vi "route.vi"() -> ()   [LabVIEW 2014]
uses:
  <vilib>/Utility/sysdir.llb/System Directory Type.ctl
  <vilib>/httpClient/LabVIEWHTTPClient.lvlib
panel:
  out "full/연료":i32
  out "time/시간":dbl
  in  "도움말":bool
  in  "피드백":bool
  in  "저장 경로":path
  out "Distance":string="0"
  in  "?":bool
  in  "?":bool
  in  "?":bool
  out "x fmc 플랜":string
  out "FMS 플랜":string
  in  "Destination":string
  in  "departure":string
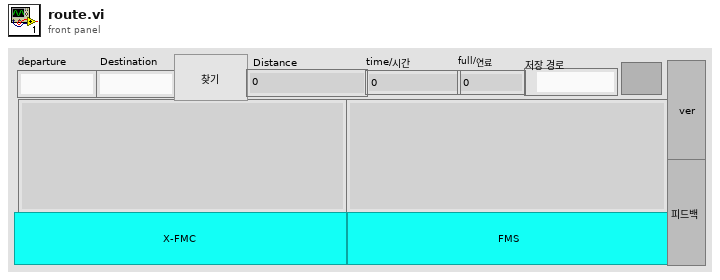
[diagram p1: front panel]
types:
  T1 = enum16{"open", "replace", "create", "open or create", "replace or create", "replace or create with confirmation"}
  T2 = typedef "System Directory Type.ctl" = i32
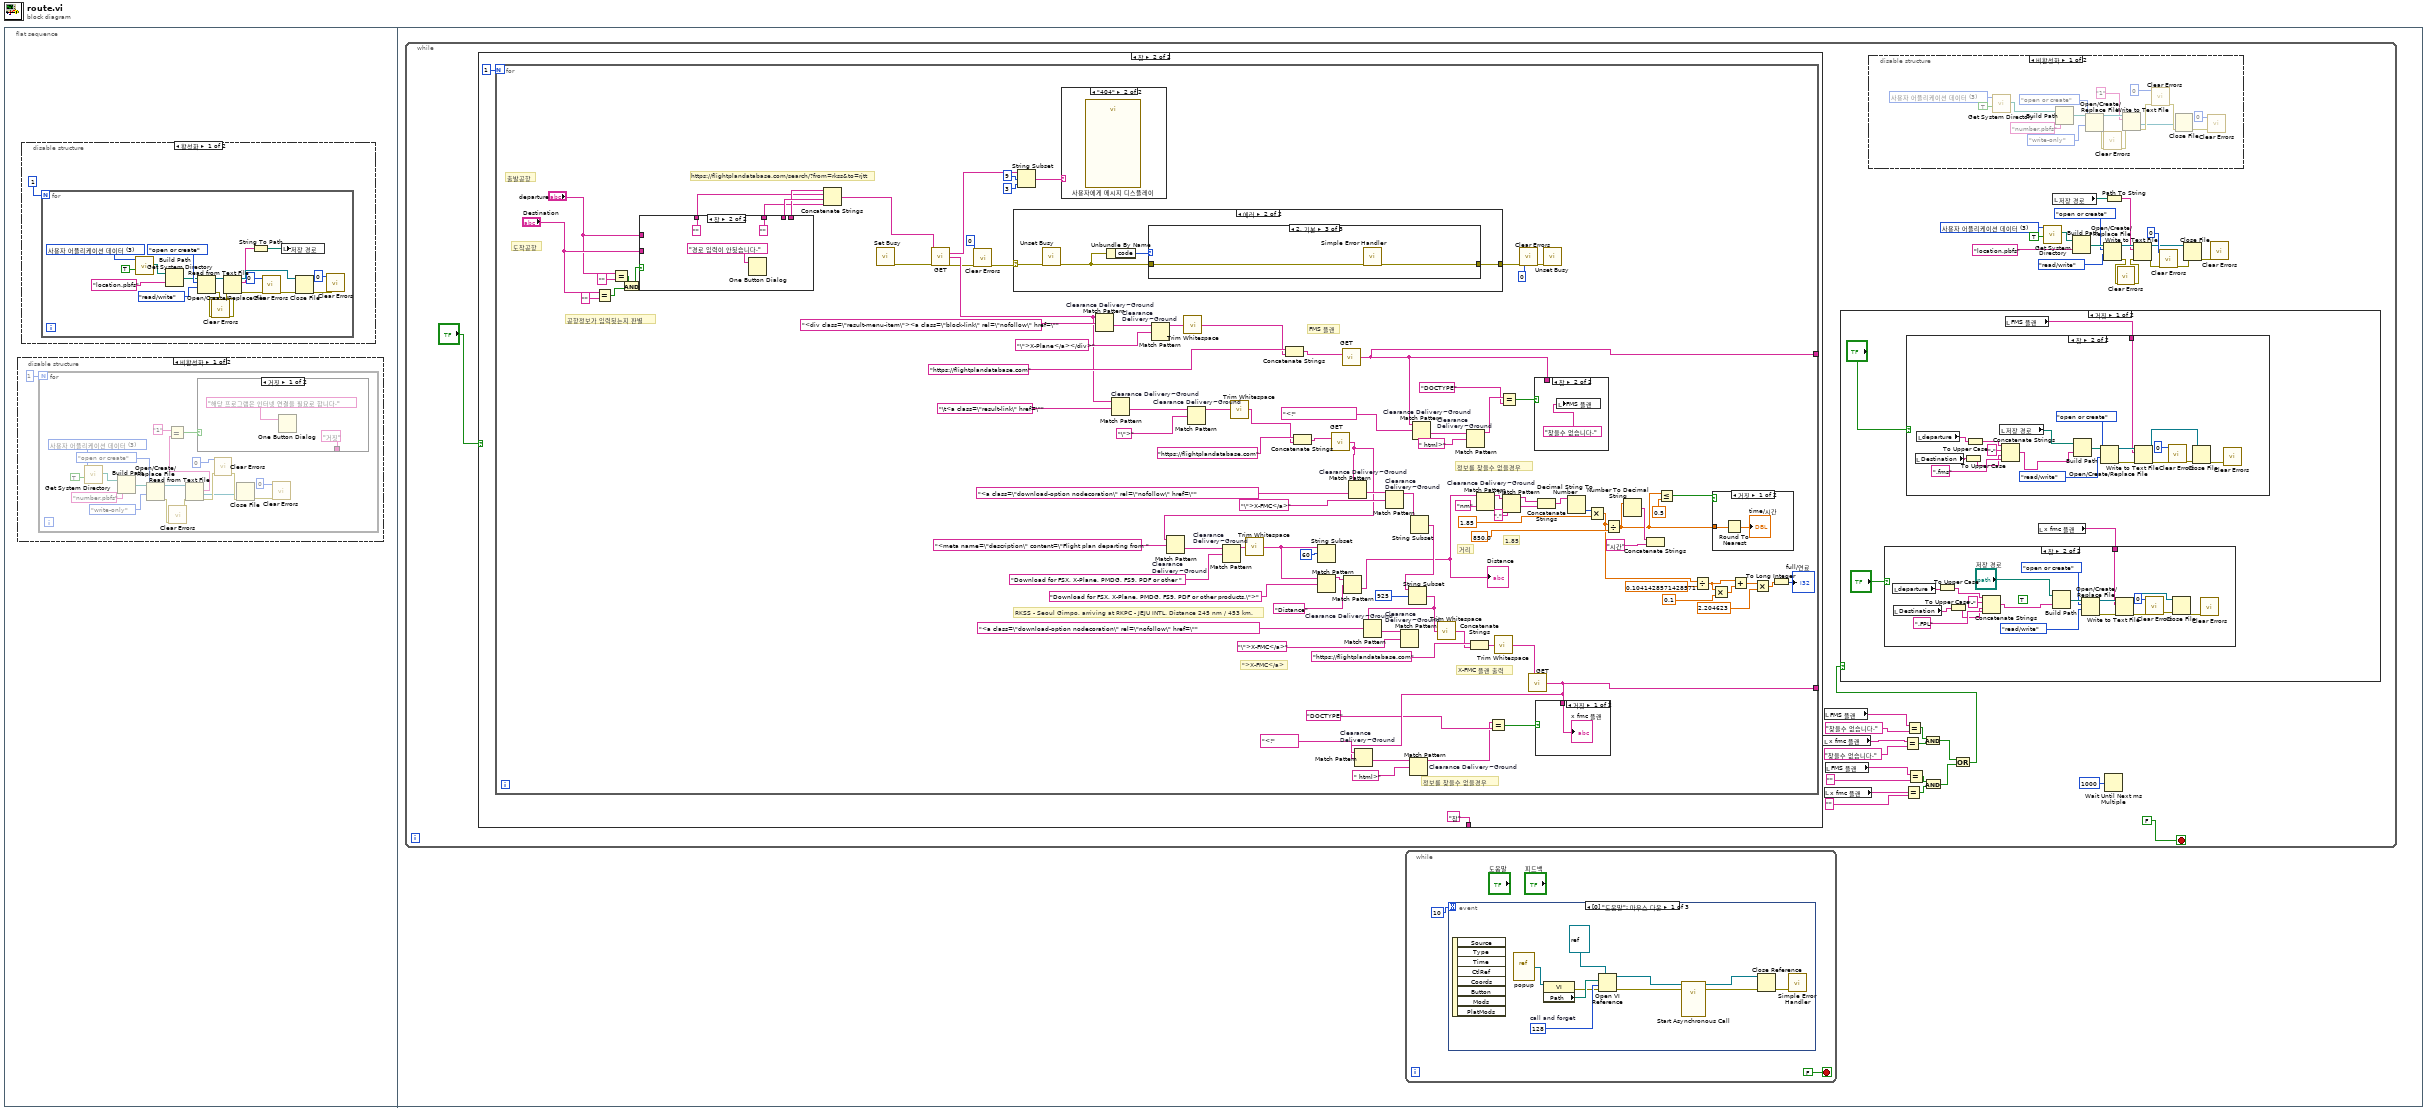
[diagram p0: block diagram]
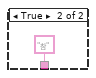
[diagram p2: hidden frame]
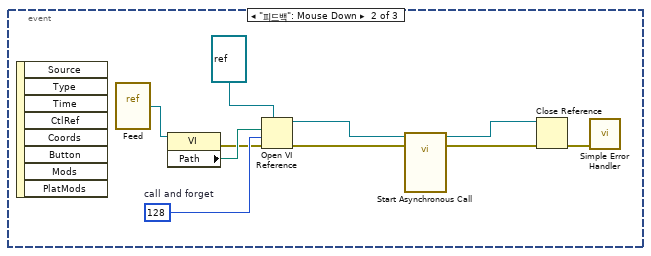
[diagram p5: hidden frame]
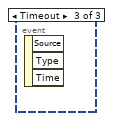
[diagram p6: hidden frame]
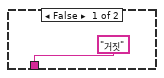
[diagram p11: hidden frame]
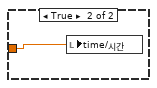
[diagram p12: hidden frame]
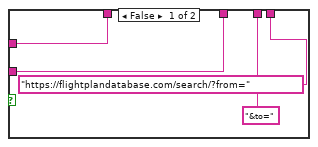
[diagram p13: hidden frame]
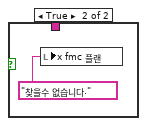
[diagram p14: hidden frame]
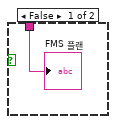
[diagram p15: hidden frame]
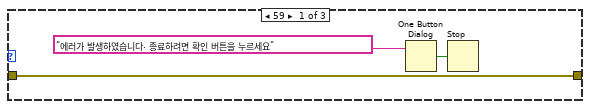
[diagram p18: hidden frame]
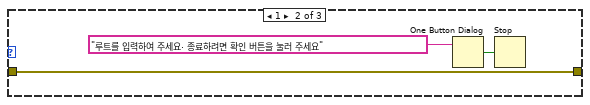
[diagram p19: hidden frame]
diagram:
  n1 = flat-sequence {
    frame #0 {
      n2 = disable-structure shown="비활성화" {
        frame Disabled {
          n3 = for {
            N: 1 -> [_]
            w7 = T2 3 items=["사용자 홈"=0, "사용자 데스크탑"=1, "사용자 문서"=2, "사용자 어플리케이션 데이터"=3, "사용자 환경"=4, "사용자 임시"=5, "퍼블릭 문서"=6, "퍼블릭 어플리케이션 데이터"=7, "퍼블릭 환경"=8, "퍼블릭 캐시"=13, "시스템 코어 라이브러리"=9, "시스템 설치된 라이브러리"=10, "어플리케이션 파일"=11, "부팅 볼륨 루트"=12] ("system directory type")
            n4 = call <vilib>:"Get System Directory.vi"("create directory if not found? (F)"=TRUE, "system directory type"=w7) -> ("system directory"=w8:path)  [unwired: 9 in]
            n5 = Build Path(base path=w8, name or relative path="number.pbfs" ("이름 또는 상대 경로")) -> (appended path=w13:path)
            n6 = Open/Create/Replace File(file path (use dialog)=w13, operation (0:open)=T1."open or create" ("동작(0:open)"), access (0:read/write)=enum16{"read/write", "read-only", "write-only"}."write-only" ("접근(0:읽기/쓰기)")) -> (refnum out=w16:refnum<file>, error out=w5:errorcluster)  [unwired: 3 in, 1 out]
            n7 = call <vilib>:"Clear Errors.vi"("error in (no error)"=w5) -> ("error out"=w4:errorcluster)  [unwired: 5 in, 1 out]
            n8 = Read from Text File(file (use dialog)=w16, error in=w4) -> (refnum out=w17:refnum<file>, text=w2:string, error out=w18:errorcluster)  [unwired: 2 in, 1 out]
            n9 = Equal?(x="1" ("y"), y=w2) -> (x = y?=w12:bool)
            n10 = case shown="거짓" w12 {
              tunnel: ["거짓" "참"] -> _
              frame False {
                n11 = One Button Dialog(message="해당 프로그램은 인터넷 연결을 필요로 합니다." ("메시지")) -> ()  [unwired: 1 in, 1 out]
              }
              frame True {
              }
            }
            n12 = call <vilib>:"Clear Errors.vi"("error in (no error)"=w18, "specific error code to clear (0: all)"=0) -> ("error out"=w19:errorcluster)  [unwired: 4 in, 1 out]
            n13 = Close File(refnum=w17, error in=w19) -> (error out=w10:errorcluster)  [unwired: 1 out]
            n14 = call <vilib>:"Clear Errors.vi"("error in (no error)"=w10, "specific error code to clear (0: all)"=0) -> ()  [unwired: 4 in, 2 out]
          }
        }
        frame Enabled {
        }
      }
      n15 = disable-structure shown="활성화" {
        frame Enabled {
          n16 = for {
            N: 1 -> [_]
            w35 = T2 3 items=["사용자 홈"=0, "사용자 데스크탑"=1, "사용자 문서"=2, "사용자 어플리케이션 데이터"=3, "사용자 환경"=4, "사용자 임시"=5, "퍼블릭 문서"=6, "퍼블릭 어플리케이션 데이터"=7, "퍼블릭 환경"=8, "퍼블릭 캐시"=13, "시스템 코어 라이브러리"=9, "시스템 설치된 라이브러리"=10, "어플리케이션 파일"=11, "부팅 볼륨 루트"=12] ("system directory type")
            n17 = call <vilib>:"Get System Directory.vi"("create directory if not found? (F)"=TRUE, "system directory type"=w35) -> ("system directory"=w36:path)  [unwired: 9 in]
            n18 = Build Path(base path=w36, name or relative path="location.pbfs" ("문자열")) -> (appended path=w39:path)
            n19 = Open/Create/Replace File(file path (use dialog)=w39, operation (0:open)=T1."open or create" ("동작(0:open)"), access (0:read/write)=enum16{"read/write", "read-only", "write-only"}."read/write" ("접근(0:읽기/쓰기)")) -> (refnum out=w25:refnum<file>, error out=w27:errorcluster)  [unwired: 3 in, 1 out]
            n20 = call <vilib>:"Clear Errors.vi"("error in (no error)"=w27) -> ("error out"=w26:errorcluster)  [unwired: 5 in, 1 out]
            n21 = Read from Text File(file (use dialog)=w25, error in=w26) -> (refnum out=w33:refnum<file>, text=w29:string, error out=w34:errorcluster)  [unwired: 2 in, 1 out]
            n22 = String To Path(string=w29) -> (path=w28:path)
            n23 = call <vilib>:"Clear Errors.vi"("error in (no error)"=w34, "specific error code to clear (0: all)"=0) -> ("error out"=w38:errorcluster)  [unwired: 4 in, 1 out]
            n24 = local write "저장 경로"(w28) -> ()
            n25 = Close File(refnum=w33, error in=w38) -> (error out=w32:errorcluster)  [unwired: 1 out]
            n26 = call <vilib>:"Clear Errors.vi"("error in (no error)"=w32, "specific error code to clear (0: all)"=0) -> ()  [unwired: 4 in, 2 out]
          }
        }
        frame Disabled {
        }
      }
    }
    frame #1 {
      n27 = while {
        stop <- FALSE stop-if-true
        w72 = T2 3 items=["사용자 홈"=0, "사용자 데스크탑"=1, "사용자 문서"=2, "사용자 어플리케이션 데이터"=3, "사용자 환경"=4, "사용자 임시"=5, "퍼블릭 문서"=6, "퍼블릭 어플리케이션 데이터"=7, "퍼블릭 환경"=8, "퍼블릭 캐시"=13, "시스템 코어 라이브러리"=9, "시스템 설치된 라이브러리"=10, "어플리케이션 파일"=11, "부팅 볼륨 루트"=12] ("system directory type")
        n28 = case shown="참" "?" {
          tunnel: ["거짓" "참"] -> _
          frame False {
          }
          frame True {
            n29 = for {
              N: 1 -> [_]
              tunnel: [w261] -> _
              tunnel: [w260] -> _
              # "1.85"
              # "RKSS - Seoul Gimpo, arriving at RKPC - JEJU INTL. Distance 245 nm / 453 km."
              # "\">X-FMC</a>"
              # "https://flightplandatabase.com/search/?from=rkss&to=rjtt"
              # "FMS 플랜"
              # "거리"
              # "X-FMC 플랜 출력"
              # "정보를 찾을수 없을경우"
              # "정보를 찾을수 없을경우"
              # "공항정보가 입력됫는지 판별"
              # "도착공항"
              # "출발공항"
              n30 = Equal?(x="Destination", y="") -> (x = y?=w197:bool)
              n31 = Equal?(x="departure", y="") -> (x = y?=w196:bool)
              n32 = And(x=w196, y=w197) -> (x .and. y?=w198:bool)
              n33 = case shown="참" w198 {
                tunnel: ["&to=" ("문자열") _] -> w187
                tunnel: ["https://flightplandatabase.com/search/?from=" ("문자열") _] -> w186
                tunnel: "Destination" -> [w266 _]
                tunnel: [w266 "" ("Destination")] -> w184
                tunnel: [w265 "" ("departure")] -> w182
                tunnel: "departure" -> [w265 _]
                frame False {
                }
                frame True {
                  n34 = One Button Dialog(message="경로 입력이 안됫습니다." ("메시지")) -> ()  [unwired: 1 in, 1 out]
                }
              }
              n35 = Concatenate Strings(w186, w182, w187, w184) -> (w250:string)
              n36 = call <vilib>:"Set Busy.vi"() -> ("error out"=w255:errorcluster)  [unwired: 10 in, 1 out]
              n37 = call <vilib>:"GET.vi"("url"=w250, "error in (no error)"=w255) -> ("headers"=w259:string, "body"=w224:string, "error out"=w207:errorcluster)  [unwired: 10 in, 1 out]
              n38 = call <vilib>:"Clear Errors.vi"("error in (no error)"=w207, "specific error code to clear (0: all)"=0) -> ("error out"=w208:errorcluster)  [unwired: 4 in, 1 out]
              n39 = case shown="에러" w208 {
                selector: w208 -> [w276 w279]
                tunnel: [w276 w277] -> w204
                frame No Error {
                }
                frame Error {
                  n40 = call <vilib>:"Unset Busy.vi"("error in (no error)"=w279) -> ("error out"=w278:errorcluster)  [unwired: 10 in]
                  n41 = Unbundle By Name(w278) -> ("code"=w280:i32)
                  n42 = case shown="2, 기본" w280 {
                    tunnel: w278 -> [w281 w286 w288]
                    tunnel: [w281 w286 w287] -> w277
                    frame 59 {
                      n43 = One Button Dialog(message="에러가 발생하였습니다. 종료하려면 확인 버튼을 누르세요" ("메시지")) -> (true=w282:bool)  [unwired: 1 in]
                      n44 = Stop(stop? (T)=w282) -> ()
                    }
                    frame 1 {
                      n45 = One Button Dialog(message="루트를 입력하여 주세요. 종료하려면 확인 버튼을 눌러 주세요" ("메시지")) -> (true=w284:bool)  [unwired: 1 in]
                      n46 = Stop(stop? (T)=w284) -> ()
                    }
                    frame 2, Default {
                      n47 = call <vilib>:"Simple Error Handler.vi"("error in (no error)"=w288) -> ("error out"=w287:errorcluster)  [unwired: 4 in, 4 out]
                    }
                  }
                }
              }
              n48 = String Subset(string=w259, offset (0)=9 ("오프셋(0)"), length (rest)=3 ("길이(나머지)")) -> (substring=w256:string)
              n49 = case shown="\"404\"" w256 {
                frame "거짓", Default {
                }
                frame "404" {
                  n50 = call "사용자에게 메시지 디스플레이"() -> ()  [unwired: 10 in, 2 out]
                }
              }
              n51 = Match Pattern "Clearance Delivery~Ground"(string=w224, regular expression="<div class=\"result-menu-item\"><a class=\"block-link\" rel=\"nofollow\" href=\"" ("정규식")) -> (after substring=w253:string)  [unwired: 1 in, 3 out]
              n52 = Match Pattern "Clearance Delivery~Ground"(string=w224, regular expression="\t<a class=\"result-link\" href=\"" ("정규식")) -> (after substring=w246:string)  [unwired: 1 in, 3 out]
              n53 = Match Pattern "Clearance Delivery~Ground"(string=w253, regular expression="\">X-Plane</a></div>" ("정규식")) -> (before substring=w251:string)  [unwired: 1 in, 3 out]
              n54 = call <vilib>:"Trim Whitespace.vi"("string"=w251) -> ("trimmed string"=w247:string)  [unwired: 1 in]
              n55 = Match Pattern "Clearance Delivery~Ground"(string=w246, regular expression="\">" ("정규식")) -> (before substring=w243:string)  [unwired: 1 in, 3 out]
              n56 = call <vilib>:"Trim Whitespace.vi"("string"=w243) -> ("trimmed string"=w241:string)  [unwired: 1 in]
              n57 = Concatenate Strings("https://flightplandatabase.com" ("url"), w247) -> (w248:string)
              n58 = Concatenate Strings("https://flightplandatabase.com" ("url"), w241) -> (w238:string)
              n59 = call <vilib>:"GET.vi"("url"=w238) -> ("body"=w222:string)  [unwired: 11 in, 3 out]
              n60 = Match Pattern "Clearance Delivery~Ground"(string=w222, regular expression="<meta name=\"description\" content=\"Flight plan departing from " ("정규식")) -> (after substring=w225:string)  [unwired: 1 in, 3 out]
              n61 = Match Pattern "Clearance Delivery~Ground"(string=w225, regular expression="Download for FSX, X-Plane, PMDG, FS9, PDF or other " ("정규식")) -> (before substring=w227:string)  [unwired: 1 in, 3 out]
              n62 = call <vilib>:"Trim Whitespace.vi"("string"=w227) -> ("trimmed string"=w192:string)  [unwired: 1 in]
              n63 = String Subset(string=w192, offset (0)=60 ("오프셋(0)")) -> ()  [unwired: 1 in, 1 out]
              n64 = Match Pattern(string=w192, regular expression="Download for FSX, X-Plane, PMDG, FS9, PDF or other products.\">" ("정규식")) -> (before substring=w190:string)  [unwired: 1 in, 3 out]
              n65 = call <vilib>:"GET.vi"("url"=w248) -> ("body"=w260:string)  [unwired: 11 in, 3 out]
              n66 = Match Pattern(string=w190, regular expression="Distance" ("정규식")) -> (after substring=w188:string)  [unwired: 1 in, 3 out]
              "Distance" <- w188
              n67 = Match Pattern "Clearance Delivery~Ground"(string=w222, regular expression="<a class=\"download-option nodecoration\" rel=\"nofollow\" href=\"" ("정규식")) -> (after substring=w237:string)  [unwired: 1 in, 3 out]
              n68 = Match Pattern "Clearance Delivery~Ground"(string=w237, regular expression="\">X-FMC</a>" ("정규식")) -> (before substring=w236:string)  [unwired: 1 in, 3 out]
              n69 = String Subset(string=w236) -> (substring=w193:string)  [unwired: 2 in]
              n70 = String Subset(string=w193, offset (0)=925 ("오프셋(0)")) -> (substring=w194:string)  [unwired: 1 in]
              n71 = Match Pattern "Clearance Delivery~Ground"(string=w194, regular expression="<a class=\"download-option nodecoration\" rel=\"nofollow\" href=\"" ("정규식")) -> (after substring=w233:string)  [unwired: 1 in, 3 out]
              n72 = Match Pattern "Clearance Delivery~Ground"(string=w233, regular expression="\">X-FMC</a>" ("정규식")) -> ()  [unwired: 1 in, 4 out]
              n73 = Match Pattern "Clearance Delivery~Ground"(string=w260, regular expression="<!" ("문자열")) -> (after substring=w219:string)  [unwired: 1 in, 3 out]
              n74 = call <vilib>:"Trim Whitespace.vi"("string"=w194) -> ("trimmed string"=w231:string)  [unwired: 1 in]
              n75 = Match Pattern "Clearance Delivery~Ground"(string=w219, regular expression=" html>" ("정규식")) -> (before substring=w218:string)  [unwired: 1 in, 3 out]
              n76 = Concatenate Strings("https://flightplandatabase.com" ("url"), w231) -> (w230:string)
              n77 = Match Pattern "Clearance Delivery~Ground"(string=w188, regular expression="nm" ("정규식")) -> (before substring=w178:string)  [unwired: 1 in, 3 out]
              n78 = call <vilib>:"Trim Whitespace.vi"("string"=w230) -> ("trimmed string"=w211:string)  [unwired: 1 in]
              n79 = Equal?(x=w218, y="DOCTYPE") -> (x = y?=w229:bool)
              n80 = Match Pattern(string=w178, regular expression="," ("정규식")) -> (before substring=w175:string, after substring=w174:string)  [unwired: 1 in, 2 out]
              n81 = call <vilib>:"Clear Errors.vi"("error in (no error)"=w204, "specific error code to clear (0: all)"=0) -> ("error out"=w205:errorcluster)  [unwired: 4 in, 1 out]
              n82 = call <vilib>:"GET.vi"("url"=w211) -> ("body"=w261:string)  [unwired: 11 in, 3 out]
              n83 = Match Pattern "Clearance Delivery~Ground"(string=w261, regular expression="<!" ("문자열")) -> (after substring=w216:string)  [unwired: 1 in, 3 out]
              n84 = Match Pattern "Clearance Delivery~Ground"(string=w216, regular expression=" html>" ("정규식")) -> (before substring=w213:string)  [unwired: 1 in, 3 out]
              n85 = Equal?(x=w213, y="DOCTYPE") -> (x = y?=w228:bool)
              n86 = case shown="참" w229 {
                tunnel: w260 -> [w274 _]
                frame False {
                  "FMS 플랜" <- w274
                }
                frame True {
                  n87 = local write "FMS 플랜"("찾을수 없습니다.") -> ()
                }
              }
              n88 = case shown="거짓" w228 {
                tunnel: w261 -> [w272 _]
                frame False {
                  "x fmc 플랜" <- w272
                }
                frame True {
                  n89 = local write "x fmc 플랜"("찾을수 없습니다.") -> ()
                }
              }
              n90 = Concatenate Strings(w175, w174) -> (w177:string)
              n91 = call <vilib>:"Unset Busy.vi"("error in (no error)"=w205) -> ()  [unwired: 10 in, 1 out]
              n92 = Decimal String To Number(string=w177) -> (number=w179:i32)  [unwired: 2 in, 1 out]
              n93 = Multiply(x=w179, y=1.85) -> (x*y=w167:dbl)
              n94 = Divide(x=w167, y=850.0) -> (x/y=w171:dbl)
              n95 = Number To Decimal String(number=w171) -> (decimal integer string=w199:string)  [unwired: 1 in]
              n96 = Concatenate Strings(w199, "시간") -> ()  [unwired: 1 out]
              n97 = Less Or Equal?(x=w171, y=0.5) -> (x <= y?=w173:bool)
              n98 = Divide(x=w167, y=0.1041428571428571) -> (x/y=w168:dbl)
              n99 = case shown="거짓" w173 {
                tunnel: w171 -> [w263 w264]
                frame False {
                  n100 = Round To Nearest(number=w263) -> (nearest integer value=→"time/시간":dbl)
                }
                frame True {
                  n101 = local write "time/시간"(w264) -> ()
                }
              }
              n102 = Multiply(x=w168, y=0.1) -> (x*y=w166:dbl)
              n103 = Add(x=w168, y=w166) -> (x+y=w165:dbl)
              n104 = Multiply(x=w165, y=2.204623) -> (x*y=w162:dbl)
              n105 = To Long Integer(number=w162) -> (32bit integer=→"full/연료":i32)
            }
          }
        }
        n106 = local read "x fmc 플랜"() -> (w95:string)
        n107 = local read "FMS 플랜"() -> (w93:string)
        n108 = local read "x fmc 플랜"() -> (w88:string)
        n109 = local read "FMS 플랜"() -> (w90:string)
        n110 = disable-structure shown="비활성화" {
          frame Disabled {
            w103 = T2 3 items=["사용자 홈"=0, "사용자 데스크탑"=1, "사용자 문서"=2, "사용자 어플리케이션 데이터"=3, "사용자 환경"=4, "사용자 임시"=5, "퍼블릭 문서"=6, "퍼블릭 어플리케이션 데이터"=7, "퍼블릭 환경"=8, "퍼블릭 캐시"=13, "시스템 코어 라이브러리"=9, "시스템 설치된 라이브러리"=10, "어플리케이션 파일"=11, "부팅 볼륨 루트"=12] ("system directory type")
            n111 = call <vilib>:"Get System Directory.vi"("create directory if not found? (F)"=TRUE, "system directory type"=w103) -> ("system directory"=w104:path)  [unwired: 9 in]
            n112 = Build Path(base path=w104, name or relative path="number.pbfs" ("이름 또는 상대 경로")) -> (appended path=w109:path)
            n113 = Open/Create/Replace File(file path (use dialog)=w109, operation (0:open)=T1."open or create" ("동작(0:open)"), access (0:read/write)=enum16{"read/write", "read-only", "write-only"}."write-only" ("접근(0:읽기/쓰기)")) -> (refnum out=w112:refnum<file>, error out=w101:errorcluster)  [unwired: 3 in, 1 out]
            n114 = call <vilib>:"Clear Errors.vi"("error in (no error)"=w101) -> ("error out"=w100:errorcluster)  [unwired: 5 in, 1 out]
            n115 = Write to Text File(file (use dialog)=w112, text="1" ("텍스트"), error in=w100) -> (refnum out=w113:refnum<file>, error out=w114:errorcluster)  [unwired: 1 in, 1 out]
            n116 = call <vilib>:"Clear Errors.vi"("error in (no error)"=w114, "specific error code to clear (0: all)"=0) -> ("error out"=w115:errorcluster)  [unwired: 4 in, 1 out]
            n117 = Close File(refnum=w113, error in=w115) -> (error out=w106:errorcluster)  [unwired: 1 out]
            n118 = call <vilib>:"Clear Errors.vi"("error in (no error)"=w106, "specific error code to clear (0: all)"=0) -> ()  [unwired: 4 in, 2 out]
          }
          frame Enabled {
          }
        }
        n119 = Equal?(x=w95, y="찾을수 없습니다.") -> (x = y?=w96:bool)
        n120 = Equal?(x=w88, y="") -> (x = y?=w66:bool)
        n121 = Equal?(x=w93, y="찾을수 없습니다.") -> (x = y?=w97:bool)
        n122 = Equal?(x=w90, y="") -> (x = y?=w87:bool)
        n123 = And(x=w97, y=w96) -> (x .and. y?=w85:bool)
        n124 = And(x=w87, y=w66) -> (x .and. y?=w86:bool)
        n125 = Or(x=w85, y=w86) -> (x .or. y?=w84:bool)
        n126 = case shown="거짓" w84 {
          frame False {
            n127 = local read "FMS 플랜"() -> (w118:string)
            n128 = case shown="참" "?" {
              tunnel: w118 -> [_ w132]
              frame False {
              }
              frame True {
                n129 = local read "Destination"() -> (w129:string)
                n130 = local read "departure"() -> (w126:string)
                n131 = To Upper Case(1:w129) -> (0:w128:string)
                n132 = To Upper Case(1:w126) -> (0:w127:string)
                n133 = local read "저장 경로"() -> (w122:path)
                n134 = Concatenate Strings(w127, "-" ("문자열"), w128, ".fms" ("문자열")) -> (w130:string)
                n135 = Build Path(base path=w122, name or relative path=w130) -> (appended path=w136:path)
                n136 = Open/Create/Replace File(file path (use dialog)=w136, operation (0:open)=T1."open or create" ("동작(0:open)"), access (0:read/write)=enum16{"read/write", "read-only", "write-only"}."read/write" ("접근(0:읽기/쓰기)")) -> (refnum out=w139:refnum<file>, error out=w138:errorcluster)  [unwired: 3 in, 1 out]
                n137 = Write to Text File(file (use dialog)=w139, text=w132, error in=w138) -> (refnum out=w137:refnum<file>, error out=w125:errorcluster)  [unwired: 1 in, 1 out]
                n138 = call <vilib>:"Clear Errors.vi"("error in (no error)"=w125, "specific error code to clear (0: all)"=0) -> ("error out"=w124:errorcluster)  [unwired: 4 in, 1 out]
                n139 = Close File(refnum=w137, error in=w124) -> (error out=w121:errorcluster)  [unwired: 1 out]
                n140 = call <vilib>:"Clear Errors.vi"("error in (no error)"=w121) -> ()  [unwired: 5 in, 2 out]
              }
            }
            n141 = local read "x fmc 플랜"() -> (w119:string)
            n142 = case shown="참" "?" {
              tunnel: w119 -> [_ w151]
              frame False {
              }
              frame True {
                (unwired) TRUE ("create directory if not found? (F)")
                n143 = local read "departure"() -> (w148:string)
                n144 = local read "Destination"() -> (w146:string)
                n145 = To Upper Case(1:w148) -> (0:w147:string)
                n146 = To Upper Case(1:w146) -> (0:w145:string)
                n147 = Concatenate Strings(w147, "-" ("문자열"), w145, ".FPL" ("문자열")) -> (w152:string)
                n148 = Build Path(base path="저장 경로", name or relative path=w152) -> (appended path=w156:path)
                n149 = Open/Create/Replace File(file path (use dialog)=w156, operation (0:open)=T1."open or create" ("동작(0:open)"), access (0:read/write)=enum16{"read/write", "read-only", "write-only"}."read/write" ("접근(0:읽기/쓰기)")) -> (refnum out=w158:refnum<file>, error out=w157:errorcluster)  [unwired: 3 in, 1 out]
                n150 = Write to Text File(file (use dialog)=w158, text=w151, error in=w157) -> (refnum out=w142:refnum<file>, error out=w144:errorcluster)  [unwired: 1 in, 1 out]
                n151 = call <vilib>:"Clear Errors.vi"("error in (no error)"=w144, "specific error code to clear (0: all)"=0) -> ("error out"=w143:errorcluster)  [unwired: 4 in, 1 out]
                n152 = Close File(refnum=w142, error in=w143) -> (error out=w140:errorcluster)  [unwired: 1 out]
                n153 = call <vilib>:"Clear Errors.vi"("error in (no error)"=w140) -> ()  [unwired: 5 in, 2 out]
              }
            }
          }
          frame True {
          }
        }
        n154 = call <vilib>:"Get System Directory.vi"("create directory if not found? (F)"=TRUE, "system directory type"=w72) -> ("system directory"=w73:path)  [unwired: 9 in]
        n155 = local read "저장 경로"() -> (w78:path)
        n156 = Build Path(base path=w73, name or relative path="location.pbfs" ("문자열")) -> (appended path=w82:path)
        n157 = Open/Create/Replace File(file path (use dialog)=w82, operation (0:open)=T1."open or create" ("동작(0:open)"), access (0:read/write)=enum16{"read/write", "read-only", "write-only"}."read/write" ("접근(0:읽기/쓰기)")) -> (refnum out=w83:refnum<file>, error out=w68:errorcluster)  [unwired: 3 in, 1 out]
        n158 = Wait Until Next ms Multiple(millisecond multiple=u32 1000 ("ms 배수")) -> ()  [unwired: 1 out]
        n159 = Path To String(path=w78) -> (string=w70:string)
        n160 = call <vilib>:"Clear Errors.vi"("error in (no error)"=w68) -> ("error out"=w67:errorcluster)  [unwired: 5 in, 1 out]
        n161 = Write to Text File(file (use dialog)=w83, text=w70, error in=w67) -> (refnum out=w74:refnum<file>, error out=w77:errorcluster)  [unwired: 1 in, 1 out]
        n162 = call <vilib>:"Clear Errors.vi"("error in (no error)"=w77, "specific error code to clear (0: all)"=0) -> ("error out"=w76:errorcluster)  [unwired: 4 in, 1 out]
        n163 = Close File(refnum=w74, error in=w76) -> (error out=w71:errorcluster)  [unwired: 1 out]
        n164 = call <vilib>:"Clear Errors.vi"("error in (no error)"=w71) -> ()  [unwired: 5 in, 2 out]
      }
      n165 = while {
        stop <- FALSE stop-if-true
        n166 = event shown="[0] \"도움말\": 마우스 다운" {
          selector: _ -> [_ _ _]
          dyn-events: _ -> [_ _ _]
          timeout: 10 -> [_ _ _]
          event "도움말": Mouse Down {
            w54 = 128  # call and forget
            n167 = event-data() -> ()  [unwired: 1 in, 8 out]
            n168 = vi-ref "popup.vi"() -> (w47:refnum<vi>)
            n169 = property class="VI"(reference=w47) -> (error out=w48:errorcluster, "Path"=w49:path)  [unwired: 1 in, 1 out]
            n170 = Open VI Reference(type specifier VI Refnum (for type only)=refnum<vi> refnum, vi path=w49, options=w54, error in (no error)=w48) -> (vi reference=w46:refnum<vi>, error out=w52:errorcluster)  [unwired: 2 in]
            n171 = call-by-ref "Start Asynchronous Call"(reference=w46, error in=w52) -> (reference out=w45:refnum<vi>, error out=w51:errorcluster)  [unwired: 12 in]
            n172 = Close Reference(reference=w45, error in (no error)=w51) -> (error out=w50:errorcluster)
            n173 = call <vilib>:"Simple Error Handler.vi"("error in (no error)"=w50) -> ()  [unwired: 4 in, 5 out]
          }
          event "피드백": Mouse Down {
            w64 = 128  # call and forget
            n174 = event-data() -> ()  [unwired: 1 in, 8 out]
            n175 = vi-ref "Feed.vi"() -> (w57:refnum<vi>)
            n176 = property class="VI"(reference=w57) -> (error out=w58:errorcluster, "Path"=w59:path)  [unwired: 1 in, 1 out]
            n177 = Open VI Reference(type specifier VI Refnum (for type only)=refnum<vi> refnum, vi path=w59, options=w64, error in (no error)=w58) -> (vi reference=w56:refnum<vi>, error out=w62:errorcluster)  [unwired: 2 in]
            n178 = call-by-ref "Start Asynchronous Call"(reference=w56, error in=w62) -> (reference out=w55:refnum<vi>, error out=w61:errorcluster)  [unwired: 12 in]
            n179 = Close Reference(reference=w55, error in (no error)=w61) -> (error out=w60:errorcluster)
            n180 = call <vilib>:"Simple Error Handler.vi"("error in (no error)"=w60) -> ()  [unwired: 4 in, 5 out]
          }
          event Timeout {
            n181 = event-data() -> ()  [unwired: 1 in, 3 out]
          }
        }
      }
    }
  }
